vi "Open API Tester.vi"(8 "error in":errorcluster, 10 "DQMH Library Ref":refnum<vi>, 11 "Application Instance":refnum<vi>) -> (0 "error out":errorcluster)   [LabVIEW 2019, in "Panther Dashboard.lvlib"]
doc: "This VI checks the Main.vi State of the selected DQMH Module"
uses:
  Panther Dashboard.lvlib
  Panther Dashboard--global.vi
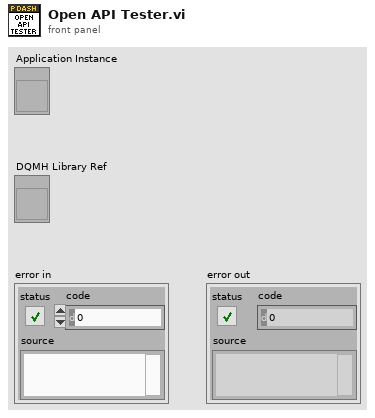
[diagram p1: front panel]
types:
  T1 = enum32{"Bad", "Idle", "Run top level", "Running"}
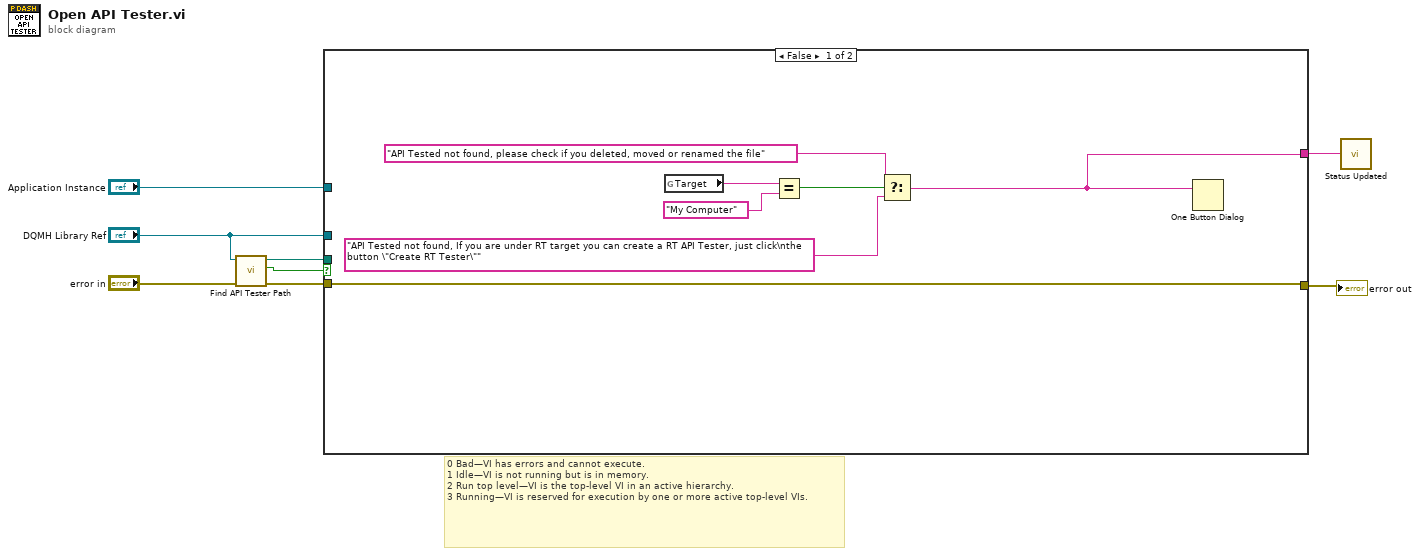
[diagram p0: block diagram]
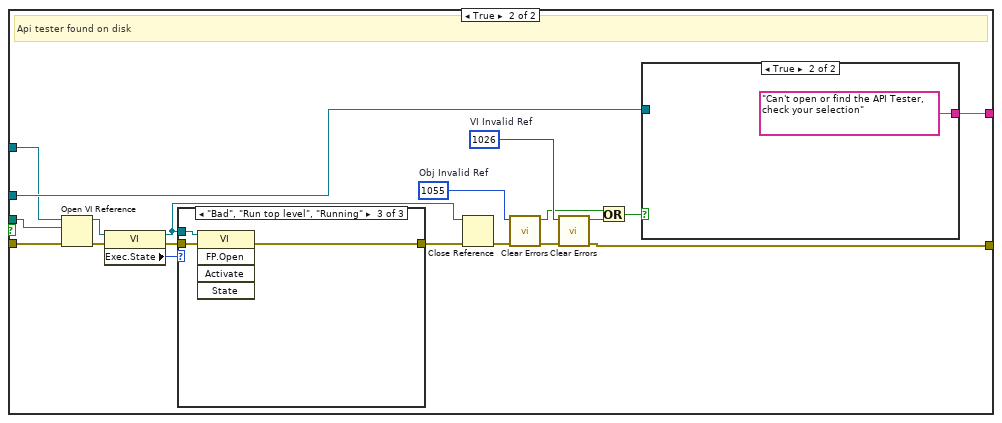
[diagram p2: hidden frame]
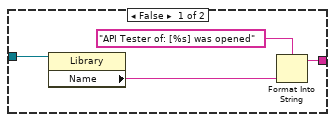
[diagram p3: hidden frame]
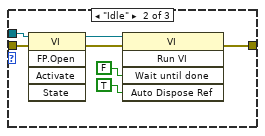
[diagram p5: hidden frame]
diagram:
  # "0\tBad—VI has errors and cannot execute.\n1\tIdle—VI is not running but is in memory.\n2\tRun top level—VI is the top-level VI in an active hierarchy.\n3\tRunning—VI is reserved for execution by one or more active top-level VIs."
  n1 = call "Find API Tester Path.vi"("error in"="error in", "DQMH Library Ref"="DQMH Library Ref") -> ("error out"=w7:errorcluster, "Api tester found?"=w2:bool, "API Tester Path"=w5:path)  [unwired: 7 in]
  n2 = case shown="False" w2 {
    tunnel: w7 -> [w15 w33]
    tunnel: w5 -> [_ w27]
    tunnel: "DQMH Library Ref" -> [_ w18]
    tunnel: "Application Instance" -> [_ w17]
    tunnel: [w15 w28] -> w6
    tunnel: [w9 w16] -> w1
    frame False {
      n3 = global read "Panther Dashboard--global.vi" "Target"() -> (w14:string)
      n4 = Equal?(x=w14, y="My Computer") -> (x = y?=w12:bool)
      n5 = Select(t="API Tested not found, please check if you deleted, moved or renamed the file", s=w12, f="API Tested not found, If you are under RT target you can create a RT API Tester, just click\nthe button \"Create RT Tester\"") -> (s? t:f=w9:string)
      n6 = One Button Dialog(message=w9) -> ()  [unwired: 1 in, 1 out]
    }
    frame True {
      w23 = 1055  # Obj Invalid Ref
      w22 = 1026  # VI Invalid Ref
      # "Api tester found on disk"
      n7 = Open VI Reference(application reference (local)=w17, vi path=w27, error in (no error)=w33) -> (vi reference=w26:refnum<vi>, error out=w34:errorcluster)  [unwired: 3 in]
      n8 = property class="VI"(reference=w26, error in=w34) -> (reference out=w24:refnum<vi>, error out=w32:errorcluster, "Exec.State"=w25:T1)
      n9 = case shown="\"Bad\", \"Run top level\", \"Running\"" w25 {
        tunnel: w24 -> [_ w41 w48]
        tunnel: w32 -> [w40 w46 w49]
        tunnel: [w40 w45 w50] -> w31
        frame Default {
        }
        frame "Idle" {
          n10 = invoke class="VI" method="FP.Open"(reference=w41, error in=w46) -> (reference out=w44:refnum<vi>, error out=w47:errorcluster)  [unwired: 3 in, 3 out]
          n11 = invoke class="VI" method="Run VI"(reference=w44, error in=w47, "Wait until done"=FALSE ("Wait Until Done"), "Auto Dispose Ref"=TRUE ("Auto Dispose Reference")) -> (error out=w45:errorcluster)  [unwired: 1 in, 4 out]
        }
        frame "Bad", "Run top level", "Running" {
          n12 = invoke class="VI" method="FP.Open"(reference=w48, error in=w49) -> (error out=w50:errorcluster)  [unwired: 3 in, 4 out]
        }
      }
      n13 = Close Reference(reference=w24, error in (no error)=w31) -> (error out=w30:errorcluster)
      n14 = call <vilib>:"Clear Errors.vi"("error in (no error)"=w30, "specific error code to clear (0: all)"=w23) -> ("error out"=w29:errorcluster, "specific error cleared?"=w21:bool)  [unwired: 4 in]
      n15 = call <vilib>:"Clear Errors.vi"("error in (no error)"=w29, "specific error code to clear (0: all)"=w22) -> ("error out"=w28:errorcluster, "specific error cleared?"=w20:bool)  [unwired: 4 in]
      n16 = Or(x=w21, y=w20) -> (x .or. y?=w19:bool)
      n17 = case shown="True" w19 {
        tunnel: w18 -> [w36 _]
        tunnel: [w35 "Can't open or find the API Tester, check your selection"] -> w16
        frame False {
          n18 = property on="Property Node" class="Library"(reference=w36) -> ("Name"=w37:string)  [unwired: 1 in, 2 out]
          n19 = Format Into String(format string="API Tester of: [%s] was opened" ("Status"), w37) -> (resulting string=w35:string)  [unwired: 2 in, 1 out]
        }
        frame True {
        }
      }
    }
  }
  "error out" <- w6
  n20 = call "Status Updated.vi"("Status"=w1) -> ()  [unwired: 10 in, 1 out]
